vi "Required String Buffer Size (Framework).vi"(8 "error in (no error)":errorcluster, 11 "Framework Configuration in":T1) -> (0 "error out":errorcluster, 2 "required string buffer size":u64 format="%d bytes", 3 "Framework Configuration out":T1)   [LabVIEW 2017, in "DSF Core.lvlib"]
uses:
  DSF Core.lvlib
  Controls/DSF Engine Framework Configuration.ctl
  Controls/DSF Engine Plugin Configuration.ctl
  Controls/DSF Timing Info.ctl
  Controls/DSF Engine Plugin Thread Configuration.ctl
  Controls/DSF Settings Info.ctl
  Controls/DSF Engine Transfer Group Configuration.ctl
  Controls/DSF Direction.ctl
  Controls/DSF Engine Transfer Configuration.ctl
  Controls/DSF Byte Order.ctl
  Controls/DSF Engine Channel Configuration.ctl
  Controls/DSF Channel Buffer Descriptor.ctl
  Controls/DSF Data Type.ctl
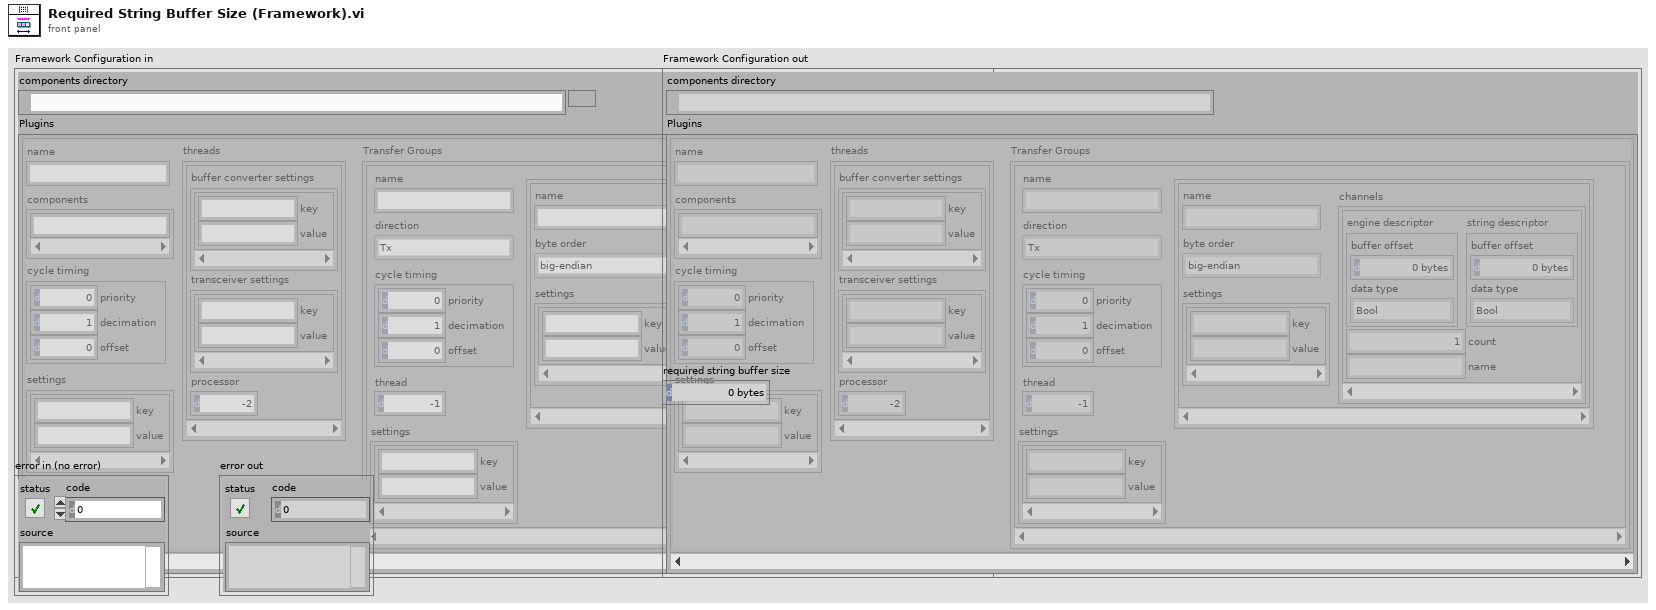
[diagram p1: front panel]
types:
  T1 = typedef "DSF Core.lvlib/DSF Engine Framework Configuration.ctl" = cluster{"components directory":path, "Plugins":T2[]}
  T2 = typedef "DSF Core.lvlib/DSF Engine Plugin Configuration.ctl" = cluster{"name":string, "components":string[], "cycle timing":T3, "threads":T4[], "Transfer Groups":T6[], "settings":T5}
  T3 = typedef "DSF Core.lvlib/DSF Timing Info.ctl" = cluster{"priority":u64, "decimation":u64, "offset":u64}
  T4 = typedef "DSF Core.lvlib/DSF Engine Plugin Thread Configuration.ctl" = cluster{"buffer converter settings":T5, "transceiver settings":T5, "processor":i32}
  T5 = typedef "DSF Core.lvlib/DSF Settings Info.ctl" = cluster{"key":string, "value":string}[]
  T6 = typedef "DSF Core.lvlib/DSF Engine Transfer Group Configuration.ctl" = cluster{"name":string, "direction":T7, "cycle timing":T3, "thread":i32, "settings":T5, "Transfers":T8[]}
  T7 = typedef "DSF Core.lvlib/DSF Direction.ctl" = enum8{"Tx", "Rx"}
  T8 = typedef "DSF Core.lvlib/DSF Engine Transfer Configuration.ctl" = cluster{"name":string, "byte order":T9, "channels":T10[], "settings":T5}
  T9 = typedef "DSF Core.lvlib/DSF Byte Order.ctl" = enum8{"big-endian", "little-endian"}
  T10 = typedef "DSF Core.lvlib/DSF Engine Channel Configuration.ctl" = cluster{"engine descriptor":T11, "string descriptor":T11, "count":u64, "name":string}
  T11 = typedef "DSF Core.lvlib/DSF Channel Buffer Descriptor.ctl" = cluster{"buffer offset":u64, "data type":T12}
  T12 = typedef "DSF Core.lvlib/DSF Data Type.ctl" = enum8{"Bool", "SGL", "DBL", "I8", "I16", "I32", "I64", "U8", "U16", "U32", "U64"}
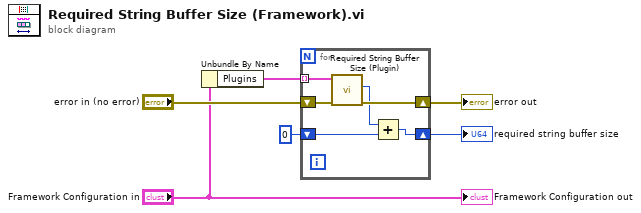
[diagram p0: block diagram]
diagram:
  n1 = Unbundle By Name("Framework Configuration in") -> ("Plugins"=w4:T2[])
  n2 = for {
    tunnel: w4 -> [w10] mode=indexing
    shift-right: [w12] -> w5
    shift-left: u64 0 -> [w11]
    shift-right: [w9] -> w2
    shift-left: "error in (no error)" -> [w8]
    n3 = call "Required String Buffer Size (Plugin).vi"("error in (no error)"=w8, "Plugin Configuration in"=w10) -> ("error out"=w9:errorcluster, "required string buffer size"=w7:u64)  [unwired: 7 in, 1 out]
    n4 = Add(x=w7, y=w11) -> (x+y=w12:u64)
  }
  "required string buffer size" <- w5
  "error out" <- w2
  "Framework Configuration out" <- "Framework Configuration in"
